vi "zxing Read Barcode.vi"(8 "error in (no error)":errorcluster, 11 "Image":T1) -> (0 "error out":errorcluster, 3 "Text":string, 5 "BarcodeFormat":i32(ring)=1 items=["AZTEC"=1, "CODABAR"=2, "CODE_39"=4, "CODE_93"=8, "CODE_128"=16, "DATA_MATRIX"=32, "EAN_8"=64, "EAN_13"=128, "ITF"=256, "MAXICODE"=512, "PDF_417"=1024, "QR_CODE"=2048, "RSS_14"=4096, "RSS_EXPANDED"=8192, "UPC_A"=16384, "UPC_E"=32768, "UPC_EAN_EXTENSION"=65536, "MSI"=131072, "All_1D"=192990, "PLESSEY"=262144])   [LabVIEW 2015]
uses:
  <vilib>/vision/Image Controls.llb/IMAQ Image.ctl
  C:/Users/a0272913/Desktop/AppRawJSON/Project/SubVI/zxing/zxing.dll
  zxing.dll
  System.Drawing
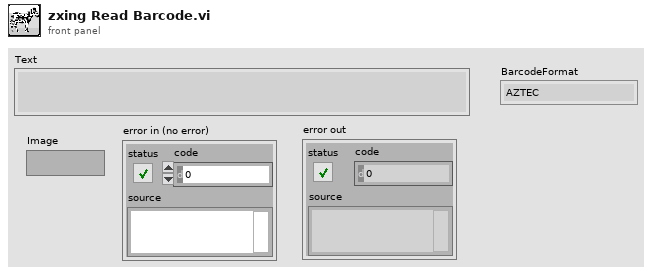
[diagram p1: front panel]
types:
  T1 = typedef "IMAQ Image.ctl" = refnum<image>
  T2 = enum32{"Map Pixel Pointer", "Unmap Pixel Pointer", "Get Pixels Infos"}
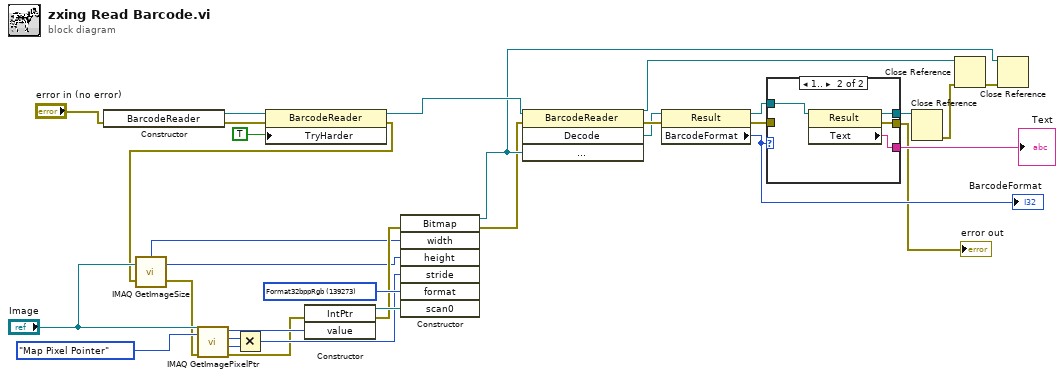
[diagram p0: block diagram]
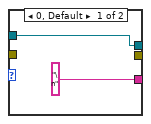
[diagram p2: hidden frame]
diagram:
  w16 = 139273 items=["DontCare, Undefined"=0, "Max"=15, "Indexed"=65536, "Gdi"=131072, "Format16bppRgb555"=135173, "Format16bppRgb565"=135174, "Format24bppRgb"=137224, "Format32bppRgb"=139273, "Format1bppIndexed"=196865, "Format4bppIndexed"=197634, "Format8bppIndexed"=198659, "Alpha"=262144, "Format16bppArgb1555"=397319, "PAlpha"=524288, "Format32bppPArgb"=925707, "Extended"=1048576, "Format16bppGrayScale"=1052676, "Format48bppRgb"=1060876, "Format64bppPArgb"=1851406, "Canonical"=2097152, "Format32bppArgb"=2498570, "Format64bppArgb"=3424269] ("format")
  n1 = constructor class="BarcodeReader"(error in="error in (no error)") -> (reference out=w32:refnum<k24>, error out=w23:errorcluster)  [unwired: 2 in, 1 out]
  n2 = property class="BarcodeReader"(reference=w32, error in=w23, "TryHarder"=TRUE) -> (reference out=w25:refnum<k24>, error out=w2:errorcluster)
  n3 = call "IMAQ GetImageSize"("Image"="Image", "error in (no error)"=w2) -> ("Y Resolution"=w9:i32, "X Resolution"=w10:i32, "error out"=w4:errorcluster)  [unwired: 2 in]
  n4 = call "IMAQ GetImagePixelPtr"("Function"=T2."Map Pixel Pointer", "error in (no error)"=w4, "Image"="Image") -> ("error out"=w3:errorcluster, "Pixel Size (Bytes)"=w13:i32, "LineWidth(Pixels)"=w14:i32, "Pixel Pointer out"=w18:u64)  [unwired: 3 in, 2 out]
  n5 = Multiply(x=w14, y=w13) -> (x*y=w12:i32)
  n6 = constructor class="IntPtr"(error in=w3, "value"=w18) -> (reference out=w15:refnum<k24>, error out=w11:errorcluster)  [unwired: 2 in, 2 out]
  n7 = constructor class="Bitmap"(error in=w11, "width"=w10, "height"=w9, "stride"=w12, "format"=w16, "scan0"=w15) -> (reference out=w7:refnum<k24>, error out=w6:errorcluster)  [unwired: 2 in, 6 out]
  n8 = invoke class="BarcodeReader" method="Decode"(reference=w25, error in=w6, "barcodeBitmap"=w7) -> (reference out=w20:refnum<k24>, error out=w31:errorcluster, "Decode"=w30:refnum<k24>)  [unwired: 1 in, 1 out]
  n9 = property class="Result"(reference=w30, error in=w31) -> (reference out=w29:refnum<k24>, error out=w28:errorcluster, "BarcodeFormat"=w26:i32)
  "BarcodeFormat" <- w26
  n10 = case shown="1.." w26 {
    tunnel: w29 -> [w33 w38]
    tunnel: w28 -> [_ _]
    tunnel: ["\n" ("Text") w37] -> w27
    tunnel: [w33 w36] -> w22
    tunnel: [_ w35] -> w1
    frame 0, Default {
    }
    frame 1.. {
      n11 = property class="Result"(reference=w38) -> (reference out=w36:refnum<k24>, error out=w35:errorcluster, "Text"=w37:string)  [unwired: 1 in]
    }
  }
  "Text" <- w27
  "error out" <- w1
  n12 = Close Reference(reference=w22) -> (error out=w21:errorcluster)  [unwired: 1 in]
  n13 = Close Reference(reference=w20, error in (no error)=w21) -> (error out=w19:errorcluster)
  n14 = Close Reference(reference=w7, error in (no error)=w19) -> ()  [unwired: 1 out]
